vi "DataHandler Start.vi"(8 "error in (no error)":errorcluster, 11 "DataLogger in":refnum<class "DataLogger.lvclass">) -> (0 "error out":errorcluster, 3 "DataLogger out":refnum<class "DataLogger.lvclass">)   [LabVIEW 2020, in "Volatus.lvlib" / "DataLogger.lvclass"]
uses:
  DataLogger.lvclass
  DataLogger.lvclass/DataLogger.ctl
  <vilib>/ActorFramework/Actor/Actor.lvclass
  DataHandler Messages/Register Groups Msg/Register Groups Msg.lvclass
  lv-promises/Promises/Promise/Promise.lvclass
  C:/dev/lv20CE/relink/lv-volatus/Volatus/DataHandlerTask/DataHandlerTask.lvclass
  C:/dev/lv20CE/relink/lv-volatus/Volatus/Task/Task.lvclass
  C:/Program Files (x86)/National Instruments/LabVIEW 2020/vi.lib/ActorFramework/Actor/Actor.lvclass
  C:/dev/lv20CE/relink/lv-volatus/Volatus/TaskStateHandler/TaskStateHandler.lvclass
  C:/dev/lv20CE/relink/lv-volatus/Volatus/VectoMessageHandler/VectoMessageHandler.lvclass
  C:/dev/lv20CE/relink/lv-volatus/Volatus/API Provider/API Provider.lvclass
  C:/dev/lv20CE/relink/lv-volatus/Volatus/DataHandler/DataHandler.lvclass
  C:/dev/lv20CE/relink/lv-volatus/Volatus/DataLogger/DataLogger.lvclass
  C:/dev/lv20CE/relink/lv-volatus/Volatus/LoggingHandler/LoggingHandler.lvclass
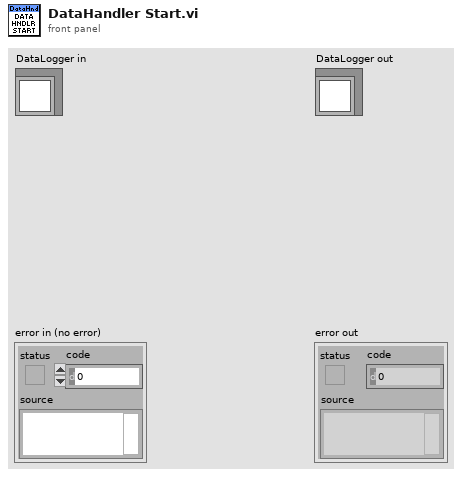
[diagram p1: front panel]
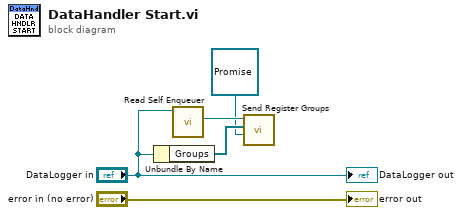
[diagram p0: block diagram]
diagram:
  n1 = Unbundle By Name("DataLogger in") -> ("Groups"=w3:refnum<class "Group.lvclass">[])
  n2 = call <vilib>:"Read Self Enqueuer.vi"("Actor"="DataLogger in") -> ("Self Enqueuer"=w4:refnum<class "Message Enqueuer.lvclass">)  [unwired: 10 in]
  n3 = call "Send Register Groups.vi"("Promise"=refnum<class "Promise.lvclass"> refnum, "Groups"=w3, "Message Enqueuer"=w4) -> ()  [unwired: 7 in, 2 out]
  "error out" <- "error in (no error)"
  "DataLogger out" <- "DataLogger in"
